vi "Conditionally Append String to Array.vi"(9 "Text to add to array":string, 10 "Append?":bool, 11 "String array in":string[](array[string])) -> (3 "String array out":string[](array[string]))   [LabVIEW 2010]
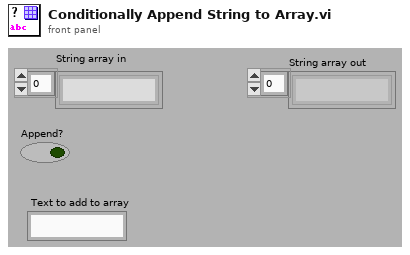
[diagram p1: front panel]
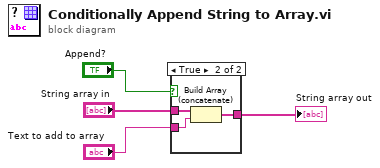
[diagram p0: block diagram]
diagram:
  n1 = case shown="True" "Append?" {
    tunnel: "Text to add to array" -> [_ w7]
    tunnel: "String array in" -> [w5 w8]
    tunnel: [w5 w6] -> w1
    frame False {
    }
    frame True {
      n2 = Build Array (concatenate)(w8, w7) -> (w6:string[])
    }
  }
  "String array out" <- w1
